vi "Create Pattern Script(Addr).vi"(8 "error in (no error)":errorcluster, 10 "Start_Addr":u16 format="%x", 11 "BML Pattern Creater in":refnum<class "BML Pattern Creater.lvclass">) -> (0 "error out":errorcluster, 2 "String":string, 3 "BML Pattern Creater out":refnum<class "BML Pattern Creater.lvclass">)   [LabVIEW 2018, in "BML Pattern Creater.lvlib" / "BML Pattern Creater.lvclass"]
uses:
  BML Pattern Creater.lvclass
  Interfaces/Protocol Interface.lvlibp/Interfaces/Protocol Interface/Pin State.ctl
  Interfaces/Protocol Interface.lvlibp/Interfaces/Protocol Interface/Protocol Interface.lvclass
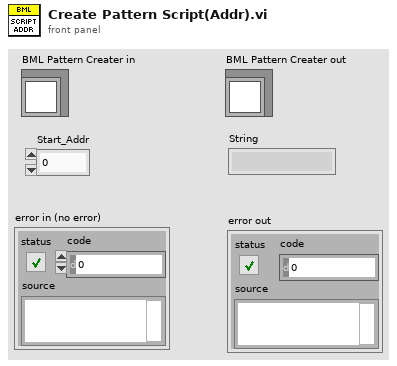
[diagram p1: front panel]
types:
  T1 = typedef "Protocol Interface.lvlibp/Protocol Interface.lvclass/Pin State.ctl" = enum16{"0", "1", "L", "H", "X", "V", "D", "M"}
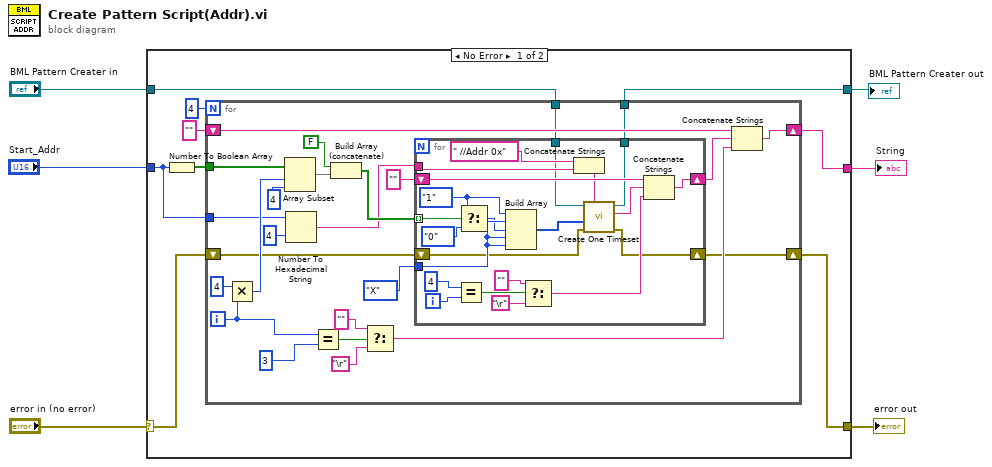
[diagram p0: block diagram]
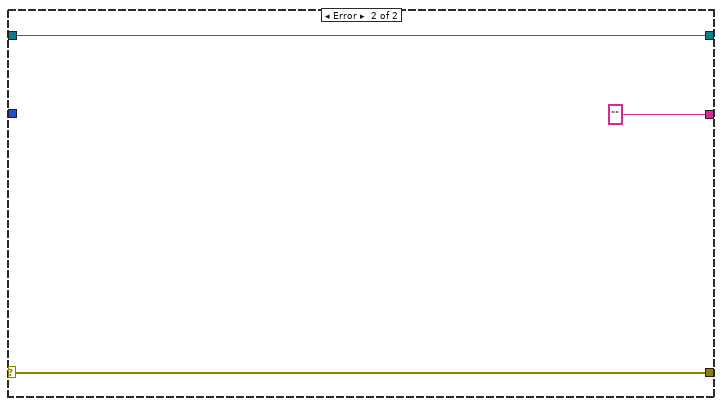
[diagram p2: hidden frame]
diagram:
  n1 = case shown="No Error" "error in (no error)" {
    selector: "error in (no error)" -> [w8 w64]
    tunnel: [w12 ""] -> w5
    tunnel: [w7 w64] -> w4
    tunnel: "Start_Addr" -> [w11 _]
    tunnel: "BML Pattern Creater in" -> [w10 w63]
    tunnel: [w9 w63] -> w1
    frame No Error {
      n2 = Number To Boolean Array(number=w11) -> (Boolean array=w15:bool[])
      n3 = for {
        N: 4 -> [_]
        tunnel: w15 -> [w40]
        shift-right: [w25] -> w12
        shift-left: "" -> [w24]
        tunnel: w11 -> [w23]
        tunnel: w10 -> [w19]
        tunnel: [w18] -> w9
        shift-right: [w17] -> w7
        shift-left: w8 -> [w16]
        i -> [w32]
        n4 = Multiply(x=4 ("y"), y=w32) -> (x*y=w38:i32)
        n5 = Array Subset(array=w40, index=w38, length=4) -> (w37:bool[])
        n6 = Number To Hexadecimal String(1:i16 4 ("width (-)"), 2:w23) -> (0:w21:string)
        n7 = Equal?(x=w32, y=3) -> (x = y?=w30:bool)
        n8 = Build Array (concatenate)(FALSE, w37) -> (w34:bool[])
        n9 = Select(t="", s=w30, f="\r") -> (s? t:f=w26:string)
        n10 = for {
          tunnel: w34 -> [w62] mode=indexing
          shift-right: [w56] -> w27
          shift-left: "" -> [w55]
          tunnel: Pin_State."X" ("PinState") -> [w53]
          tunnel: w21 -> [w50]
          tunnel: w19 -> [w45]
          tunnel: [w44] -> w18
          shift-right: [w42] -> w17
          shift-left: w16 -> [w41]
          i -> [w61]
          w49 = Pin_State."1" ("PinState")
          n11 = Equal?(x=4, y=w61) -> (x = y?=w59:bool)
          n12 = Select(t=w49, s=w62, f=Pin_State."0" ("PinState")) -> (s? t:f=w52:T1)
          n13 = Build Array(w49, w53, w52, w53, w53) -> (w46:T1[])
          n14 = Select(t="", s=w59, f="\r") -> (s? t:f=w54:string)
          n15 = Concatenate Strings(" //Addr 0x" ("Notes"), w50) -> (w47:string)
          n16 = call-dynamic "Create One Timeset.vi"("Notes"=w47, "error in (no error)"=w41, "Pin State"=w46, "BML Pattern Creater in"=w45) -> ("error out"=w42:errorcluster, "string out"=w43:string, "BML Pattern Creater out"=w44:refnum<class "BML Pattern Creater.lvclass">)  [unwired: 5 in]
          n17 = Concatenate Strings(w55, w43, w54) -> (w56:string)
        }
        n18 = Concatenate Strings(w24, w27, w26) -> (w25:string)
      }
    }
    frame Error {
    }
  }
  "String" <- w5
  "error out" <- w4
  "BML Pattern Creater out" <- w1
